vi "Initialize Tree.vi"(8 "error in":errorcluster, 11 "Module Data":T1) -> (0 "error out":errorcluster, 3 "Module Data":T1)   [LabVIEW 2020, in "Peek Window.lvlib"]
uses:
  Peek Window.lvlib
  MHL Data Cluster.ctl
  Open Diagram Argument--cluster.ctl
  Symbols Enum.ctl
  cb685dd4-87ab-4bc3-90dd-f8513bb521dc.vi
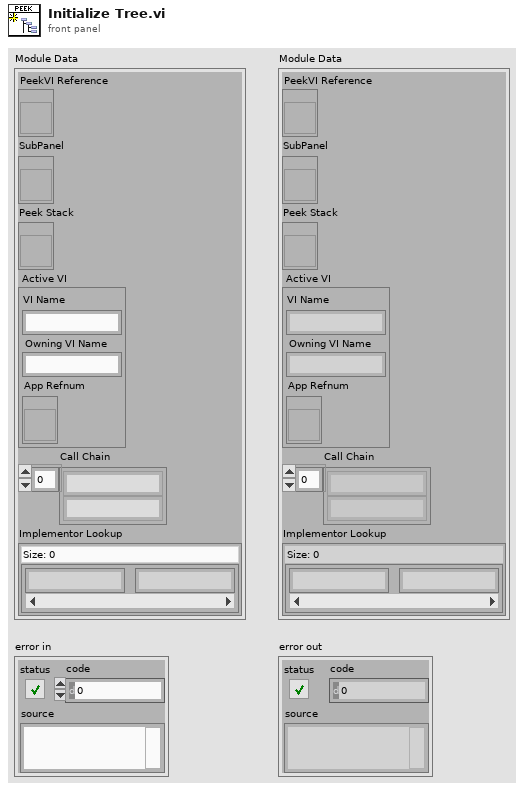
[diagram p1: front panel]
types:
  T1 = typedef "Peek Window.lvlib/MHL Data Cluster.ctl" = cluster{"PeekVI Reference":refnum<vi>, "SubPanel":refnum<vi>, "Peek Stack":refnum<vi>, "Active VI":T2, "Call Chain":string[], "Implementor Lookup":map{string, string}}
  T2 = typedef "Peek Window.lvlib/Open Diagram Argument--cluster.ctl" = cluster{"VI Name":string, "Owning VI Name":string, "App Refnum":refnum<vi>}
  T3 = typedef "Peek Window.lvlib/Symbols Enum.ctl" = enum16{"<Blank>", "Below Here Glyph", "VI", "Dynamic Dispatch VI"}
  T4 = typedef "imagedata.ctl" = cluster{"image type":i32, "image depth":i32, "image":u8[], "mask":u8[], "colors":u32[], "Rectangle":cluster{"left":i16, "top":i16, "right":i16, "bottom":i16}}
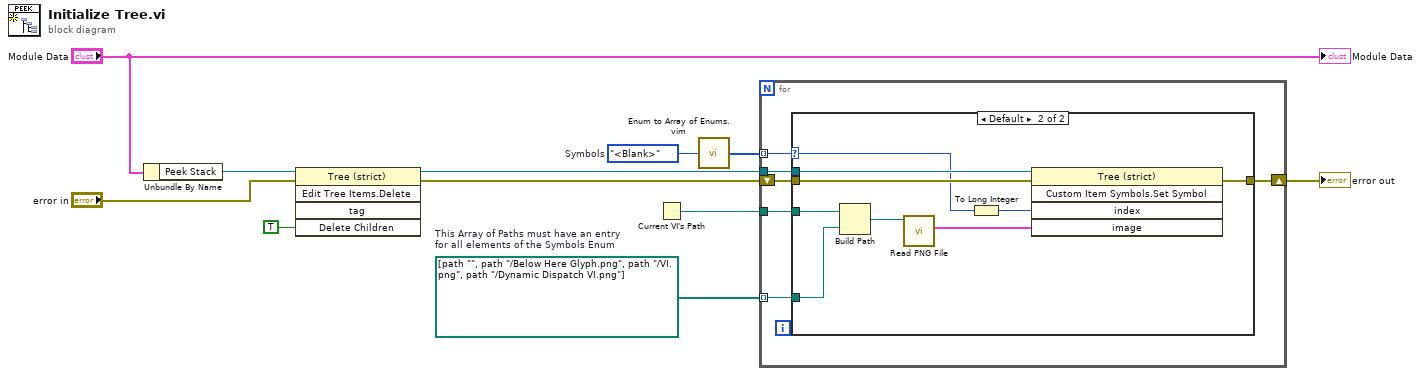
[diagram p0: block diagram]
diagram:
  w4 = Symbols_Enum."<Blank>"  # Symbols
  w1 = path[] [path "", path "../Below Here Glyph.png", path "../VI.png", path "../Dynamic Dispatch VI.png"]  # This Array of Paths must have an entry for all elements of the Symbols Enum
  n1 = Unbundle By Name("Module Data") -> ("Peek Stack"=w11:refnum<vi>)
  n2 = invoke class="Tree (strict)" method="Edit Tree Items.Delete"(reference=w11, error in="error in", "Delete Children"=TRUE ("Delete Children?")) -> (reference out=w9:refnum<vi>, error out=w8:errorcluster)  [unwired: 2 in, 3 out]
  n3 = Current VI's Path() -> (path=w5:path)
  n4 = call "Enum to Array of Enums.vim"("enum"=w4) -> ("array of enums"=w2:T3[])
  n5 = for {
    tunnel: w9 -> [w17]
    tunnel: w5 -> [w15]
    shift-right: [w14] -> w3
    shift-left: w8 -> [w16]
    tunnel: w2 -> [w13] mode=indexing
    tunnel: w1 -> [w12] mode=indexing
    n6 = case shown="Default" w13 {
      selector: w13 -> [_ w20]
      tunnel: w17 -> [_ w27]
      tunnel: w16 -> [w18 w26]
      tunnel: w15 -> [_ w23]
      tunnel: [w18 w22] -> w14
      tunnel: w12 -> [_ w21]
      frame "<Blank>" {
      }
      frame Default {
        n7 = Build Path(base path=w23, name or relative path=w21) -> (appended path=w25:path)
        n8 = call <vilib>:"Read PNG File.vi"("path to PNG file"=w25) -> ("image data"=w24:T4)  [unwired: 8 in, 2 out]
        n9 = To Long Integer(number=w20) -> (32bit integer=w19:i32)
        n10 = invoke class="Tree (strict)" method="Custom Item Symbols.Set Symbol"(reference=w27, error in=w26, "index"=w19, "image"=w24) -> (error out=w22:errorcluster)  [unwired: 1 in, 4 out]
      }
    }
  }
  "error out" <- w3
  "Module Data" <- "Module Data"
